vi "Configurate Serial Communication Settings.vi"() -> (0 "STOP ALL 2":bool, 1 "Exit and Reload":bool)   [LabVIEW 2016]
uses:
  Typedef/Serial_config_cluster.ctl
panel:
  in  "Load Button":bool
  in  "STOP ALL":bool
  in  "Exit and Reload":bool
  in  "EXIT":bool
  in  "Save Button":bool
  in  "Cluster":T1={"Termination Character"=10, "End Read on"=TRUE, "VISA resource name"="COM1", "baud rate"=9600, "data bits"=8, "parity"=enum."None", "stop bits"=10, "flow control"=0, "XON"=enum."DC1", "XOFF"=enum."DC3", "End Write on"=TRUE} {"Termination Character" format="%.0x"; "flow control" items=["None"=0, "XON/XOFF"=1, "RTS/CTS"=2, "DTR/DSR"=4]; "data bits" min=5 max=8 step=1; "stop bits" items=["1.0"=10, "1.5"=15, "2.0"=20]; "baud rate" items=["75"=75, "110"=110, "134"=134, "150"=150, "300"=300, "600"=600, "1200"=1200, "1800"=1800, "2400"=2400, "4800"=4800, "7200"=7200, "9600"=9600, "14400"=14400, "19200"=19200, "28800"=28800, "38400"=38400, "56000"=56000, "57600"=57600, "115200"=115200, "128000"=128000, "230400"=230400]}
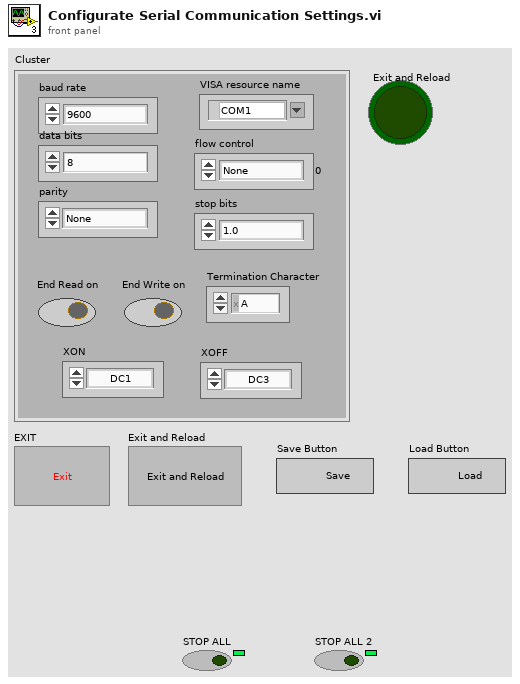
[diagram p1: front panel]
types:
  T1 = typedef "Serial_config_cluster.ctl" = cluster{"Termination Character":u8, "End Read on":bool, "VISA resource name":refnum<visa-resource-name>, "baud rate":u32, "data bits":u16, "parity":enum16{"None", "Odd", "Even", "Mark", "Space"}, "stop bits":u16, "flow control":u16, "XON":enum16{"NUL", "SOH", "STX", "ETX", "EOT", "ENQ", "ACK", "BEL", "BS", "HT", "LF", "VT", "FF", "CR", "SO", "SI", "DLE", "DC1", "DC2", "DC3", "DC4", "NAK", "SYN", "ETB", "CAN", "EM", "SUB", "ESC", "FS", "GS", "RS", "US", "SP", "!", "\"", "#", "$", "%", "&", "'", "(", ")", "*", "+", ",", "- (-)", ".", "/", "0", "1", "2", "3", "4", "5", "6", "7", "8", "9", ":", ";", "<", "=", ">", "?", "@", "A", "B", "C", "D", "E", "F", "G", "H", "I", "J", "K", "L", "M", "N", "O", "P", "Q", "R", "S", "T", "U", "V", "W", "X", "Y", "Z", "[", "\\", "]", "^", "_", "`", "a", "b", "c", "d", "e", "f", "g", "h", "i", "j", "k", "l", "m", "n", "o", "p", "q", "r", "s", "t", "u", "v", "w", "x", "y", "z", "{", "|", "}", "~"}, "XOFF":enum16{"NUL", "SOH", "STX", "ETX", "EOT", "ENQ", "ACK", "BEL", "BS", "HT", "LF", "VT", "FF", "CR", "SO", "SI", "DLE", "DC1", "DC2", "DC3", "DC4", "NAK", "SYN", "ETB", "CAN", "EM", "SUB", "ESC", "FS", "GS", "RS", "US", "SP", "!", "\"", "#", "$", "%", "&", "'", "(", ")", "*", "+", ",", "- (-)", ".", "/", "0", "1", "2", "3", "4", "5", "6", "7", "8", "9", ":", ";", "<", "=", ">", "?", "@", "A", "B", "C", "D", "E", "F", "G", "H", "I", "J", "K", "L", "M", "N", "O", "P", "Q", "R", "S", "T", "U", "V", "W", "X", "Y", "Z", "[", "\\", "]", "^", "_", "`", "a", "b", "c", "d", "e", "f", "g", "h", "i", "j", "k", "l", "m", "n", "o", "p", "q", "r", "s", "t", "u", "v", "w", "x", "y", "z", "{", "|", "}", "~"}, "End Write on":bool}
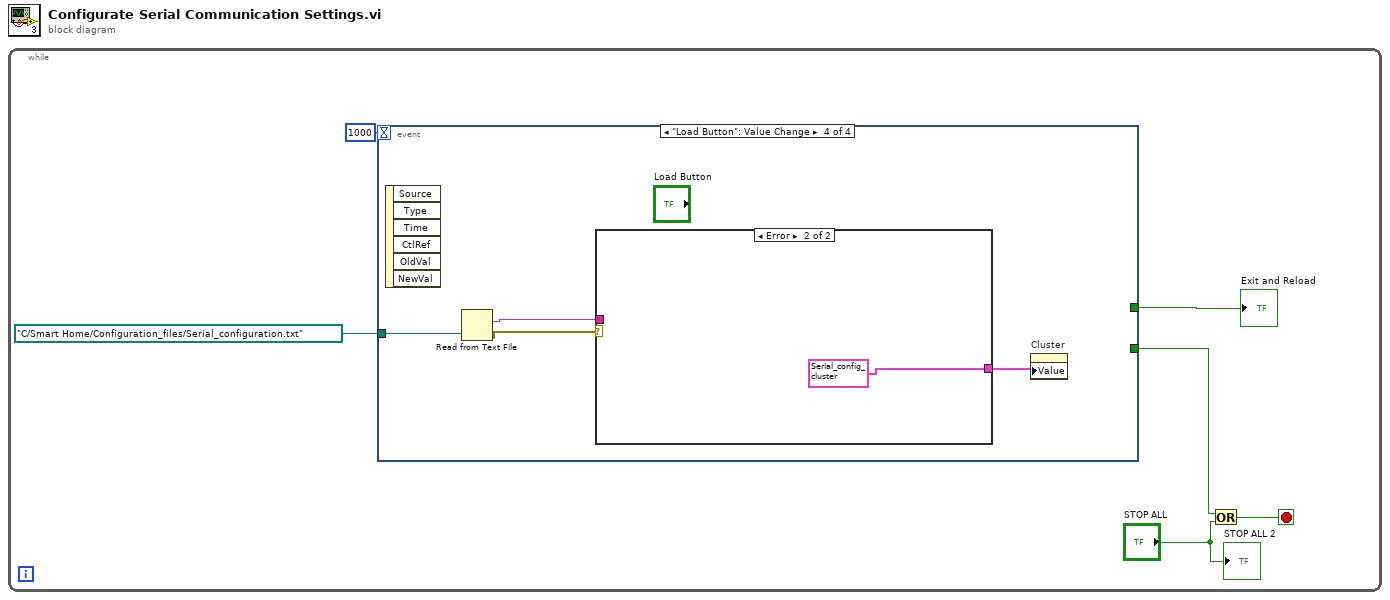
[diagram p0: block diagram]
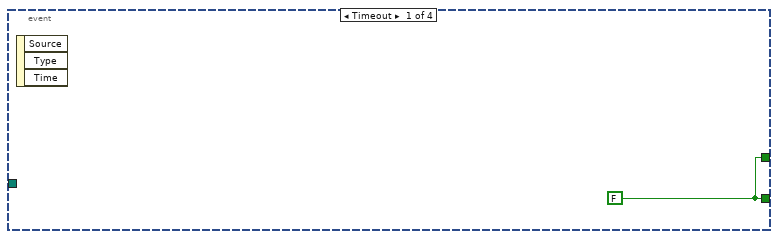
[diagram p2: hidden frame]
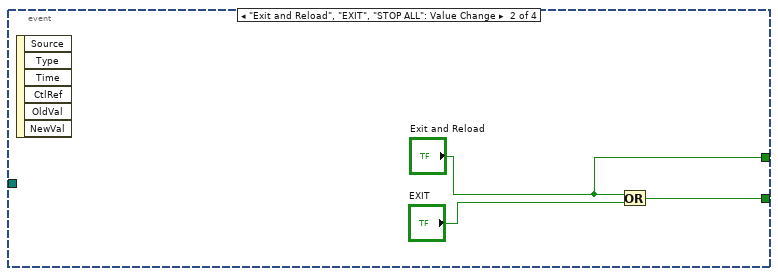
[diagram p3: hidden frame]
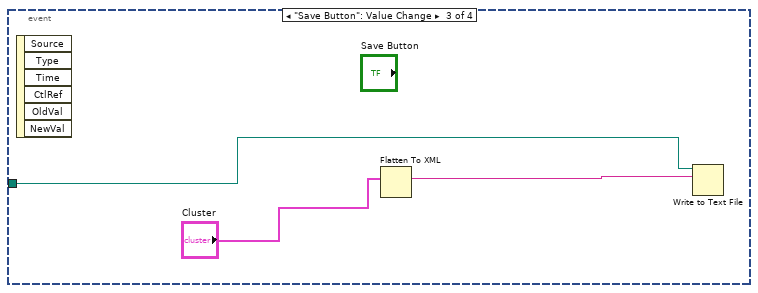
[diagram p4: hidden frame]
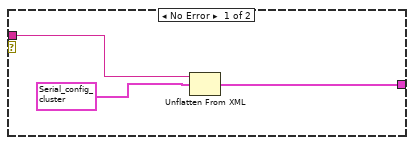
[diagram p5: hidden frame]
diagram:
  n1 = while {
    stop <- w4 stop-if-true
    n2 = event shown="[3] \"Load Button\": Value Change" {
      selector: _ -> [_ _ _ _]
      dyn-events: _ -> [_ _ _ _]
      timeout: 1000 -> [_ _ _ _]
      tunnel: [w7 w9 _ _] -> w3
      tunnel: [w7 "Exit and Reload" _ _] -> w5
      tunnel: path "C:/Smart Home/Configuration_files/Serial_configuration.txt" ("file (use dialog)") -> [_ _ w11 w17]
      event Timeout {
        w7 = FALSE
        n3 = event-data() -> ()  [unwired: 1 in, 3 out]
      }
      event "Exit and Reload", "EXIT", "STOP ALL": Value Change {
        n4 = event-data() -> ()  [unwired: 1 in, 6 out]
        n5 = Or(x="Exit and Reload", y="EXIT") -> (x .or. y?=w9:bool)
      }
      event "Save Button": Value Change {
        n6 = event-data() -> ()  [unwired: 1 in, 6 out]
        n7 = Flatten To XML(anything="Cluster") -> (xml string=w12:string)
        n8 = Write to Text File(file (use dialog)=w11, text=w12) -> ()  [unwired: 2 in, 3 out]
      }
      event "Load Button": Value Change {
        n9 = event-data() -> ()  [unwired: 1 in, 6 out]
        n10 = Read from Text File(file (use dialog)=w17) -> (text=w15:string, error out=w16:errorcluster)  [unwired: 3 in, 2 out]
        n11 = case shown="Error" w16 {
          tunnel: w15 -> [w19 _]
          tunnel: [w18 T1 {"Termination Character"=10, "End Read on"=TRUE, "VISA resource name"="COM1", "baud rate"=9600, "data bits"=6, "parity"=enum."None", "stop bits"=10, "flow control"=0, "XON"=enum."DC1", "XOFF"=enum."DC3", "End Write on"=TRUE} ("Cluster 2")] -> w14
          frame No Error {
            n12 = Unflatten From XML(xml string=w19, type=T1 {"Termination Character"=10, "End Read on"=TRUE, "VISA resource name"="COM1", "baud rate"=9600, "data bits"=6, "parity"=enum."None", "stop bits"=10, "flow control"=0, "XON"=enum."DC1", "XOFF"=enum."DC3", "End Write on"=TRUE} ("Cluster 2")) -> (value=w18:T1)  [unwired: 1 in, 1 out]
          }
          frame Error {
          }
        }
        n13 = property on="Cluster" class="Clust (strict)"("Value"=w14) -> ()  [unwired: 2 in, 2 out]
      }
    }
    "Exit and Reload" <- w5
    n14 = Or(x=w3, y="STOP ALL") -> (x .or. y?=w4:bool)
    "STOP ALL 2" <- "STOP ALL"
  }
